vi "Set RHS.vi"(8 "error in (no error)":errorcluster, 10 "RHS":variant, 11 "RHS_2D_Numeric in":refnum<class "NI_RHS_2D_Numeric.lvclass">) -> (0 "error out":errorcluster, 3 "RHS_2D_Numeric out":refnum<class "NI_RHS_2D_Numeric.lvclass">)   [LabVIEW 2017, in "NI_PDE.lvlib" / "NI_RHS_2D_Numeric.lvclass"]
uses:
  <vilib>/gmath/pde.llb/RHSClass/RHS_2D_Numeric/NI_RHS_2D_Numeric.lvclass
  <vilib>/gmath/pde.llb/RHSClass/RHS_2D_Numeric/NI_RHS_2D_Numeric.lvclass/NI_RHS_2D_Numeric.ctl
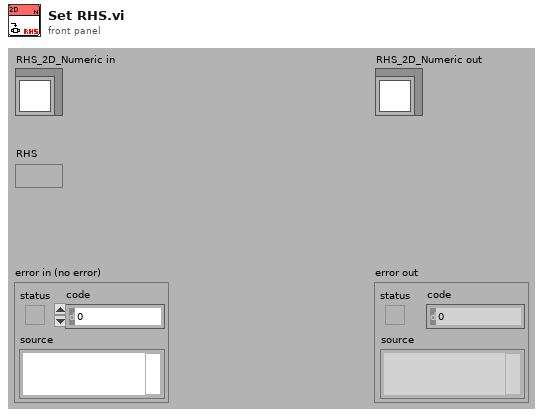
[diagram p1: front panel]
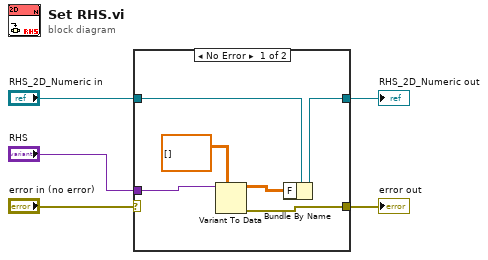
[diagram p0: block diagram]
diagram:
  n1 = case shown="No Error" "error in (no error)" {
    selector: "error in (no error)" -> [_ w13]
    tunnel: "RHS_2D_Numeric in" -> [w9 w12]
    tunnel: [w8 w12] -> w5
    tunnel: [w6 w13] -> w4
    tunnel: "RHS" -> [w11 _]
    frame No Error {
      n2 = Variant To Data(type=dbl[][] [] ("F"), Variant=w11) -> (data=w7:dbl[][], error out=w6:errorcluster)  [unwired: 1 in]
      n3 = Bundle By Name(cluster=w9, "F"=w7) -> (w8:refnum<class "NI_RHS_2D_Numeric.lvclass">)
    }
    frame Error {
    }
  }
  "RHS_2D_Numeric out" <- w5
  "error out" <- w4
